vi "MGI RWA INI Tag Lookup.vi"(10 "String":string, 11 "State In":T1={"StrToSpecifiedText"=variant, "Specified Data"=variant, "Float Fmt"="%#_13g", "Major Vers"=0, "Options"={"TS Fmt"="", "Int Fmt"="", "Delimiter"=","}}) -> (1 "INI Text":string, 2 "Text Found?":bool, 3 "State Out":T1={"StrToSpecifiedText"=variant, "Specified Data"=variant, "Float Fmt"="%#_13g", "Major Vers"=0, "Options"={"TS Fmt"="", "Int Fmt"="", "Delimiter"=","}})   [LabVIEW 2016]
doc: "Look for the specified tag in the Read Anything File. If not found, the tag is looked for in the Default Data of the variant.\n\nAuthored by Shawn Walpole\nsupport@mooregoodideas.com\nwww.mooregoodideas.com\n\nCopyright (c) 2010, Moore Good Ideas, Inc.\n\nAll rights reserved.\n\nRedistribution and use in source and binary forms, with or without modification, are permitted provided that the following conditions are met:\n\n * Redistributions of source code must retain the above copyright notice, this list of conditions and the following disclaimer.\n * Redistributions in binary form must reproduce the above copyright notice, this list of conditions and the following disclaimer in the documentation and/or other materials provided with the distribution.\n * Neither the name of Moore Good Ideas, Inc. nor the names of its contributors may be used to endorse or promote products derived from this software without specific prior written permission.\n\nTHIS SOFTWARE IS PROVIDED BY THE COPYRIGHT HOLDERS AND CONTRIBUTORS \"AS IS\" AND ANY EXPRESS OR IMPLIED WARRANTIES, INCLUDING, BUT NOT LIMITED TO, THE IMPLIED WARRANTIES OF MERCHANTABILITY AND FITNESS FOR A PARTICULAR PURPOSE ARE DISCLAIMED. IN NO EVENT SHALL THE COPYRIGHT OWNER OR CONTRIBUTORS BE LIABLE FOR ANY DIRECT, INDIRECT, INCIDENTAL, SPECIAL, EXEMPLARY, OR CONSEQUENTIAL DAMAGES (INCLUDING, BUT NOT LIMITED TO, PROCUREMENT OF SUBSTITUTE GOODS OR SERVICES; LOSS OF USE, DATA, OR PROFITS; OR BUSINESS INTERRUPTION) HOWEVER CAUSED AND ON ANY THEORY OF LIABILITY, WHETHER IN CONTRACT, STRICT LIABILITY, OR TORT (INCLUDING NEGLIGENCE OR OTHERWISE) ARISING IN ANY WAY OUT OF THE USE OF THIS SOFTWARE, EVEN IF ADVISED OF THE POSSIBILITY OF SUCH DAMAGE."
uses:
  <userlib>/_MGI/Read Write Anything/MGI RWA Tag Lookup Cluster.ctl
  <userlib>/_MGI/Read Write Anything/MGI RWA Options Cluster.ctl
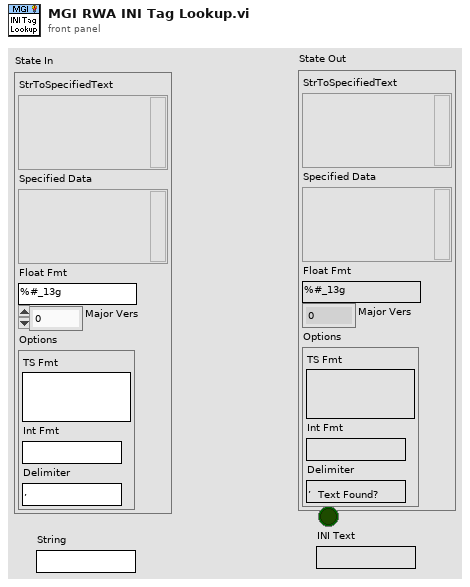
[diagram p1: front panel]
types:
  T1 = typedef "MGI RWA Tag Lookup Cluster.ctl" = cluster{"StrToSpecifiedText":variant, "Specified Data":variant, "Float Fmt":string, "Major Vers":i32, "Options":T2}
  T2 = typedef "MGI RWA Options Cluster.ctl" = cluster{"TS Fmt":string, "Int Fmt":string, "Delimiter":string}
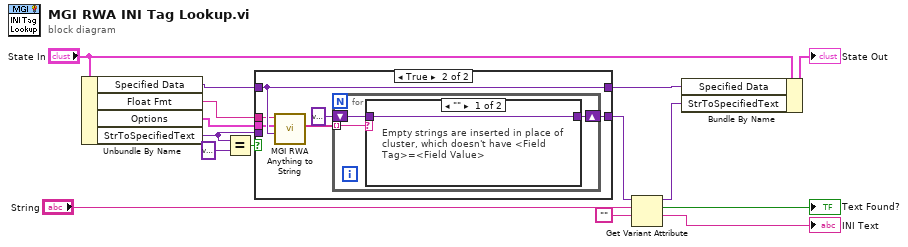
[diagram p0: block diagram]
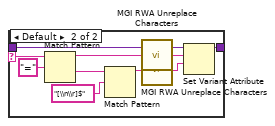
[diagram p3: hidden frame]
diagram:
  n1 = Unbundle By Name("State In") -> ("Specified Data"=w1:variant, "Float Fmt"=w9:string, "Options"=w8:T2, "StrToSpecifiedText"=w3:variant)
  n2 = Equal?(x=w3, y=variant ("StrToDefault Variant")) -> (x = y?=w6:bool)
  n3 = case shown="True" w6 {
    tunnel: w3 -> [w16 _]
    tunnel: w1 -> [w17 w23]
    tunnel: [w17 w23] -> w11
    tunnel: [w16 w21] -> w5
    tunnel: w9 -> [_ w19]
    tunnel: w8 -> [_ w18]
    frame False {
    }
    frame True {
      n4 = call <userlib>:"MGI RWA Anything to String.vi"("Anything"=w23, "Read/Write Options"=w18, "Format String (%#_13g)"=w19) -> ("Strings[]"=w20:string[])  [unwired: 1 in, 7 out]
      n5 = for {
        shift-right: [w25] -> w21
        shift-left: variant ("variant") -> [w26]
        tunnel: w20 -> [w24] mode=indexing
        n6 = case shown="\"\"" w24 {
          selector: w24 -> [_ w28]
          tunnel: w26 -> [w27 w36]
          tunnel: [w27 w35] -> w25
          frame "" {
            # "Empty strings are inserted in place of cluster, which doesn't have <Field Tag>=<Field Value>"
          }
          frame Default {
            n7 = Match Pattern(string=w28, regular expression="=") -> (before substring=w34:string, after substring=w31:string)  [unwired: 3 out]
            n8 = Match Pattern(string=w31, regular expression="[\\n\\r]$") -> (before substring=w30:string)  [unwired: 4 out]
            n9 = call <userlib>:"MGI RWA Unreplace Characters.vi"("String In"=w34) -> ("String Out"=w33:string)  [unwired: 1 out]
            n10 = call <userlib>:"MGI RWA Unreplace Characters.vi"("String In"=w30) -> ("String Out"=w32:string)  [unwired: 1 out]
            n11 = Set Variant Attribute(Variant=w36, name=w33, value=w32) -> (Variant out=w35:variant)  [unwired: 1 in, 2 out]
          }
        }
      }
    }
  }
  n12 = Get Variant Attribute(Variant=w5, name="String", default value (empty Variant)="") -> (duplicate Variant=w2:variant, found=→"Text Found?":bool, value=→"INI Text":string)  [unwired: 1 in, 1 out]
  n13 = Bundle By Name(cluster="State In", "Specified Data"=w11, "StrToSpecifiedText"=w2) -> (→"State Out":T1)
